vi "SIC.vi"(0 "System no.":i32=1 min=1 max=4 step=1, 1 "Analog input ID":i32=1 min=1 max=10 step=1, 2 "Calculation type":i32 min=0 step=1, 3 "Parameter":dbl[](array[numeric]), 4 "No. of digits":i16=4, 5 "error in":errorcluster) -> (14 "Controller error":bool, 19 "error out":errorcluster)   [LabVIEW 2026]
doc: "Set fast alignment input calculation.\nCalculation type:\n0 = Calculation OFF\n1 = Exponential Calculation \nCalculated Input Signal = Parameter0 + Parameter1 * Parameter2^(Parameter3*Voltage)\n2 = Polynomial Calculation\n Calculated Input Signal = Parameter0 + Parameter1*Voltage^1 + Parameter2*Voltage^2 + Parameter3*Voltage^3 + Parameter4*Voltage^4)\n\nC-887, E-712: \nE-727: Only calculation type 0 supported."
panel:
  # "Set fast alignment Input Calculation"
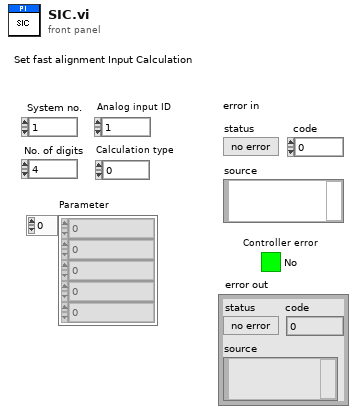
[diagram p1: front panel]
types:
  T1 = enum16{"Disable error check", "Force error check", "Use global settings"}
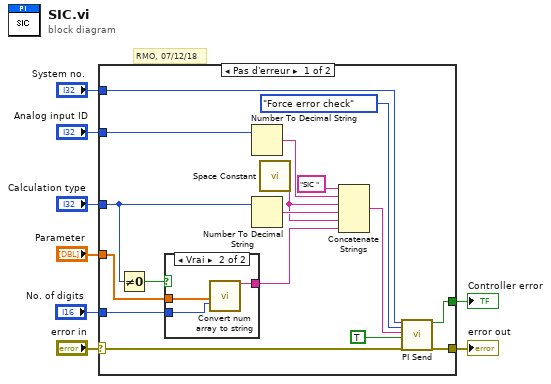
[diagram p0: block diagram]
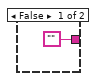
[diagram p2: hidden frame]
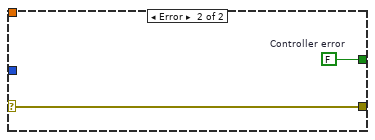
[diagram p3: hidden frame]
diagram:
  # "RMO, 07/12/18"
  n1 = case shown="Pas d'erreur" "error in" {
    selector: "error in" -> [w21 w31]
    tunnel: [w11 w31] -> w8
    tunnel: "Analog input ID" -> [w24 _]
    tunnel: "System no." -> [w19 _]
    tunnel: "Parameter" -> [w18 _]
    tunnel: "No. of digits" -> [w17 _]
    tunnel: "Calculation type" -> [w12 _]
    tunnel: [w10 w30] -> w1
    frame No Error {
      n2 = Not Equal To 0?(x=w12) -> (x != 0?=w13:bool)
      n3 = case shown="Vrai" w13 {
        tunnel: w18 -> [_ w29]
        tunnel: w17 -> [_ w28]
        tunnel: ["" w27] -> w16
        frame False {
        }
        frame True {
          n4 = call "Convert num array to string.vi"("Num. values"=w29, "No. of digits"=w28) -> ("Output string"=w27:string)  [unwired: 17 out]
        }
      }
      n5 = Number To Decimal String(number=w24) -> (decimal integer string=w22:string)  [unwired: 1 out]
      n6 = Number To Decimal String(number=w12) -> (decimal integer string=w15:string)  [unwired: 1 out]
      n7 = call <vilib>:"Space Constant.vi"() -> ("String"=w14:string)
      n8 = Concatenate Strings("SIC ", w22, w14, w15, w14, w16) -> (w23:string)
      n9 = call "PI Send.vi"("System no."=w19, "Error check settings"=T1."Force error check", "String to send"=w23, "Attach termination char.?"=TRUE ("Attach Linefeed?"), "error in"=w21) -> ("Controller error"=w10:bool, "error out"=w11:errorcluster)  [unwired: 1 in, 12 out]
    }
    frame Error {
      w30 = FALSE  # Controller error
    }
  }
  "error out" <- w8
  "Controller error" <- w1
